vi "BaseProvider_RandomWireConfig.vi"(0 "EdgeColor":refnum<vi>, 1 "_CenterThickness":refnum<vi>, 2 "_EdgeThickness":refnum<vi>, 3 "_CenterColor2":refnum<vi>, 4 "_CenterColor1":refnum<vi>, 6 "_CenterPattern":refnum<vi>, 8 "_TunnelsAndTerminalsColors":refnum<vi>) -> ()   [LabVIEW 2020]
uses:
  <resource>/Framework/Providers/Open_GDS/ClassProviders/Common/LvIcon_class/GDSLvIcon_ColorControl.ctl
  <resource>/Framework/Providers/Open_GDS/SubVIs/GOOP_WirePattern.ctl
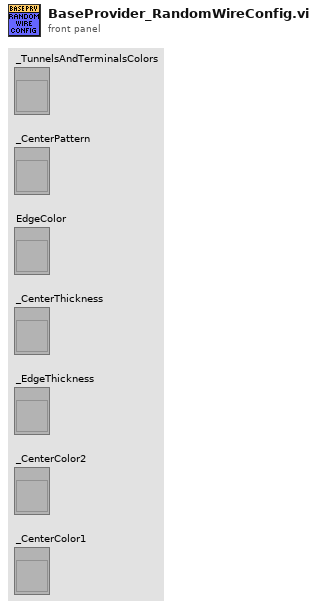
[diagram p1: front panel]
types:
  T1 = typedef "GDSLvIcon_ColorControl.ctl" = cluster{"Decal":bool, "Color":u32}
  T2 = enum16{"0 pixels", "1 pixel", "2 pixels", "3 pixels"}
  T3 = enum16{"1 pixel", "2 pixels", "3 pixels", "4 pixels", "5 pixels"}
  T4 = typedef "GOOP_WirePattern.ctl" = enum16{"Solid", "Large dash", "Small dash"}
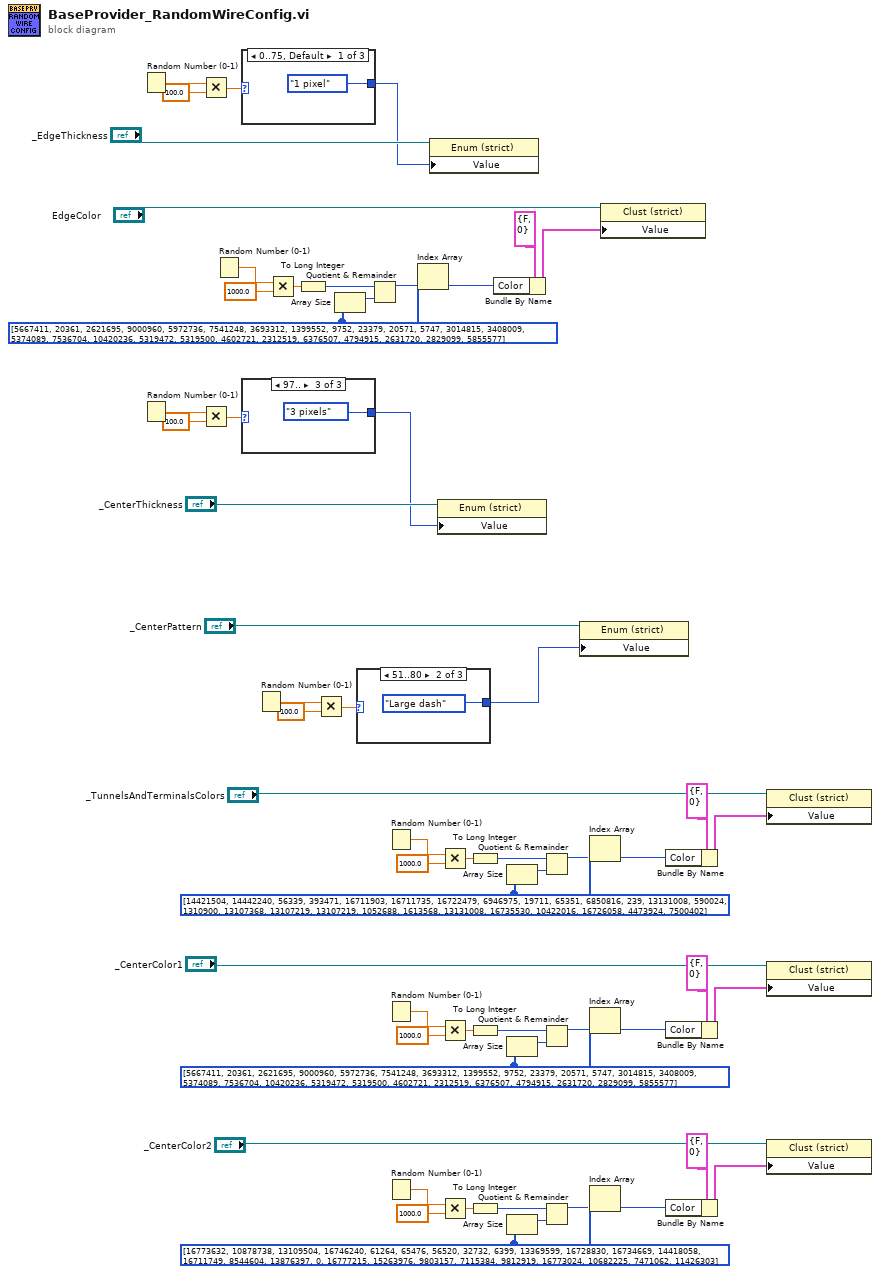
[diagram p0: block diagram]
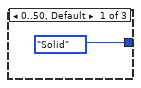
[diagram p2: hidden frame]
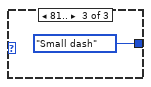
[diagram p3: hidden frame]
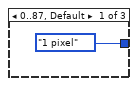
[diagram p4: hidden frame]
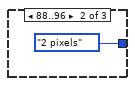
[diagram p5: hidden frame]
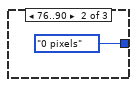
[diagram p6: hidden frame]
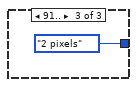
[diagram p7: hidden frame]
diagram:
  w9 = u32[] [16773632, 10878738, 13109504, 16746240, 61264, 65476, 56520, 32732, 6399, 13369599, 16728830, 16734669, 14418058, 16711749, 8544604, 13876397, 0, 16777215, 15263976, 9803157, 7115384, 9812919, 16773024, 10682225, 7471062, 11426303]
  w16 = u32[] [5667411, 20361, 2621695, 9000960, 5972736, 7541248, 3693312, 1399552, 9752, 23379, 20571, 5747, 3014815, 3408009, 5374089, 7536704, 10420236, 5319472, 5319500, 4602721, 2312519, 6376507, 4794915, 2631720, 2829099, 5855577]
  w30 = u32[] [14421504, 14442240, 56339, 393471, 16711903, 16711735, 16722479, 6946975, 19711, 65351, 6850816, 239, 13131008, 590024, 1310900, 13107368, 13107219, 13107219, 1052688, 1613568, 13131008, 16735530, 10422016, 16726058, 4473924, 7500402]
  w49 = u32[] [5667411, 20361, 2621695, 9000960, 5972736, 7541248, 3693312, 1399552, 9752, 23379, 20571, 5747, 3014815, 3408009, 5374089, 7536704, 10420236, 5319472, 5319500, 4602721, 2312519, 6376507, 4794915, 2631720, 2829099, 5855577]
  n1 = Random Number (0-1)() -> (number: 0 to 1=w58:dbl)
  n2 = Random Number (0-1)() -> (number: 0 to 1=w41:dbl)
  n3 = Multiply(x=w58, y=100.0) -> (x*y=w56:dbl)
  n4 = Multiply(x=w41, y=100.0) -> (x*y=w43:dbl)
  n5 = Random Number (0-1)() -> (number: 0 to 1=w53:dbl)
  n6 = case shown="0..75, Default" w56 {
    tunnel: [T2."1 pixel" ("Value") T2."0 pixels" ("Value") T2."2 pixels" ("Value")] -> w55
    frame 0..75, Default {
    }
    frame 76..90 {
    }
    frame 91.. {
    }
  }
  n7 = case shown="97.." w43 {
    tunnel: [T3."1 pixel" ("Value") T3."2 pixels" ("Value") T3."3 pixels" ("Value")] -> w38
    frame 0..87, Default {
    }
    frame 88..96 {
    }
    frame 97.. {
    }
  }
  n8 = Random Number (0-1)() -> (number: 0 to 1=w37:dbl)
  n9 = Multiply(x=w53, y=1000.0) -> (x*y=w52:dbl)
  n10 = To Long Integer(number=w52) -> (32bit integer=w48:i32)
  n11 = Multiply(x=w37, y=100.0) -> (x*y=w35:dbl)
  n12 = Array Size(array=w49) -> (size(s)=w51:i32)
  n13 = case shown="51..80" w35 {
    tunnel: [GOOP_WirePattern."Solid" ("Value") GOOP_WirePattern."Large dash" ("Value") GOOP_WirePattern."Small dash" ("Value")] -> w34
    frame 0..50, Default {
    }
    frame 51..80 {
    }
    frame 81.. {
    }
  }
  n14 = Quotient & Remainder(x=w48, y=w51) -> (x-y*floor(x/y)=w50:i32)  [unwired: 1 out]
  n15 = Random Number (0-1)() -> (number: 0 to 1=w26:dbl)
  n16 = Random Number (0-1)() -> (number: 0 to 1=w20:dbl)
  n17 = Random Number (0-1)() -> (number: 0 to 1=w5:dbl)
  n18 = Index Array(array=w49, index=w50) -> (element=w45:u32)
  n19 = property class="Enum (strict)"(reference="_EdgeThickness", "Value"=w55) -> ()  [unwired: 1 in, 2 out]
  n20 = property class="Enum (strict)"(reference="_CenterThickness", "Value"=w38) -> ()  [unwired: 1 in, 2 out]
  n21 = Multiply(x=w26, y=1000.0) -> (x*y=w27:dbl)
  n22 = Multiply(x=w20, y=1000.0) -> (x*y=w19:dbl)
  n23 = Multiply(x=w5, y=1000.0) -> (x*y=w6:dbl)
  n24 = To Long Integer(number=w27) -> (32bit integer=w31:i32)
  n25 = To Long Integer(number=w19) -> (32bit integer=w15:i32)
  n26 = To Long Integer(number=w6) -> (32bit integer=w10:i32)
  n27 = Bundle By Name(cluster=T1 {"Decal"=FALSE, "Color"=0} ("Value"), "Color"=w45) -> (w44:T1)
  n28 = Array Size(array=w30) -> (size(s)=w28:i32)
  n29 = Array Size(array=w16) -> (size(s)=w18:i32)
  n30 = Array Size(array=w9) -> (size(s)=w7:i32)
  n31 = Quotient & Remainder(x=w31, y=w28) -> (x-y*floor(x/y)=w29:i32)  [unwired: 1 out]
  n32 = Quotient & Remainder(x=w15, y=w18) -> (x-y*floor(x/y)=w17:i32)  [unwired: 1 out]
  n33 = Quotient & Remainder(x=w10, y=w7) -> (x-y*floor(x/y)=w8:i32)  [unwired: 1 out]
  n34 = property class="Enum (strict)"(reference="_CenterPattern", "Value"=w34) -> ()  [unwired: 1 in, 2 out]
  n35 = Index Array(array=w30, index=w29) -> (element=w33:u32)
  n36 = Index Array(array=w16, index=w17) -> (element=w13:u32)
  n37 = Index Array(array=w9, index=w8) -> (element=w12:u32)
  n38 = property class="Clust (strict)"(reference="EdgeColor", "Value"=w44) -> ()  [unwired: 1 in, 2 out]
  n39 = Bundle By Name(cluster=T1 {"Decal"=FALSE, "Color"=0} ("Value"), "Color"=w33) -> (w23:T1)
  n40 = Bundle By Name(cluster=T1 {"Decal"=FALSE, "Color"=0} ("Value"), "Color"=w13) -> (w22:T1)
  n41 = Bundle By Name(cluster=T1 {"Decal"=FALSE, "Color"=0} ("Value"), "Color"=w12) -> (w3:T1)
  n42 = property class="Clust (strict)"(reference="_TunnelsAndTerminalsColors", "Value"=w23) -> ()  [unwired: 1 in, 2 out]
  n43 = property class="Clust (strict)"(reference="_CenterColor1", "Value"=w22) -> ()  [unwired: 1 in, 2 out]
  n44 = property class="Clust (strict)"(reference="_CenterColor2", "Value"=w3) -> ()  [unwired: 1 in, 2 out]
